vi "Jog Single Step.vi"(8 "error in (no error)":errorcluster, 10 "Jog Direction":T1, 11 "Axis in":refnum<class "Axis.lvclass">) -> (0 "error out":errorcluster, 3 "Axis out":refnum<class "Axis.lvclass">)   [LabVIEW 2018, in "Axis.lvlib" / "Axis.lvclass"]
doc: "Commands the Axis to jog the specified direction in a single step size."
uses:
  Axis.lvclass
  Custom Controls/Jog Direction.ctl
  Axis.lvlib
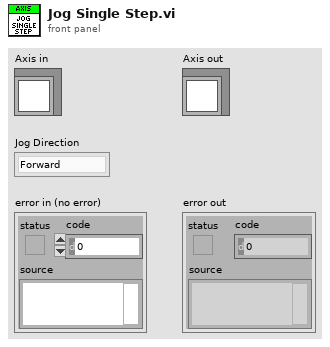
[diagram p1: front panel]
types:
  T1 = typedef "Axis.lvlib/Jog Direction.ctl" = enum16{"Forward", "Backward"}
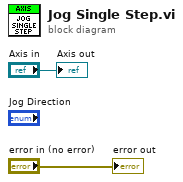
[diagram p0: block diagram]
diagram:
  "error out" <- "error in (no error)"
  "Axis out" <- "Axis in"
